vi "Get Helium Level.vi"(8 "error in (no error)":errorcluster, 11 "instrument.PPMS in":refnum<class "instrument.PPMS1.lvclass">) -> (0 "error out":errorcluster, 2 "LHe Level (%)":dbl, 3 "instrument.PPMS out":refnum<class "instrument.PPMS1.lvclass">)   [LabVIEW 2016, in "instrument.PPMS1.lvclass"]
uses:
  instrument.PPMS1.lvclass
  Typedefs/PPMS1.Commands-enum.ctl
panel:
  in  "Data":variant
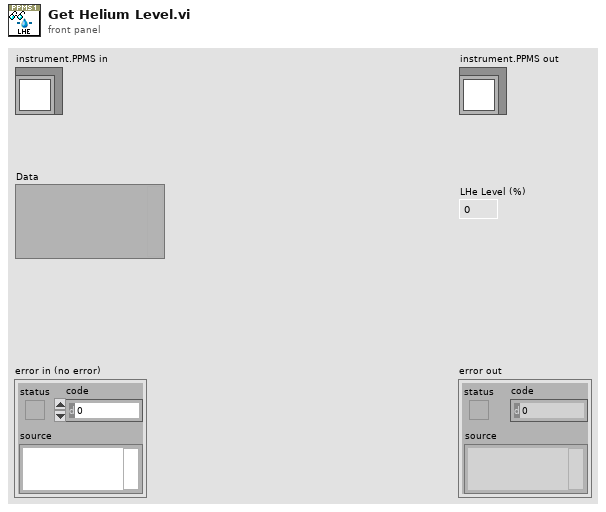
[diagram p1: front panel]
types:
  T1 = typedef "instrument.PPMS1.lvclass/PPMS1.Commands-enum.ctl" = enum16{"Get Magnet Field", "Get Helium Level", "Get Temperature", "Set Magnet Field", "Set Temperature", "getAll"}
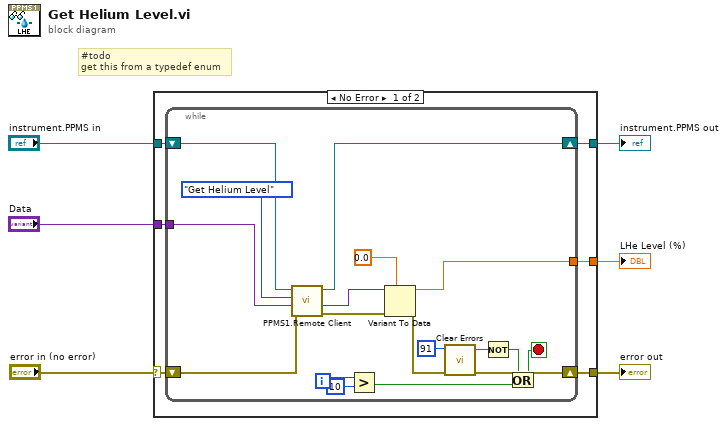
[diagram p0: block diagram]
diagram:
  # "#todo\nget this from a typedef enum"
  n1 = case shown="No Error" "error in (no error)" {
    selector: "error in (no error)" -> [w9 w32]
    tunnel: [w7 _] -> w6
    tunnel: "Data" -> [w12 _]
    tunnel: "instrument.PPMS in" -> [w11 w31]
    tunnel: [w8 w32] -> w3
    tunnel: [w10 w31] -> w2
    frame No Error {
      n2 = while {
        tunnel: w12 -> [w28]
        tunnel: [w19] -> w7
        shift-right: [w23] -> w10
        shift-left: w11 -> [w25]
        shift-right: [w21] -> w8
        shift-left: w9 -> [w22]
        i -> [w17]
        stop <- w15 stop-if-true
        n3 = call "PPMS1.Remote Client.vi"("error in (no error)"=w22, "Data"=w28, "Command"=PPMS1.Commands-enum."Get Helium Level", "instrument.PPMS in"=w25) -> ("error out"=w29:errorcluster, "Data out"=w26:variant, "instrument.PPMS out"=w23:refnum<class "instrument.PPMS1.lvclass">)  [unwired: 4 in, 1 out]
        n4 = Greater?(x=w17, y=10) -> (0:w13:bool)
        n5 = Variant To Data(error in=w29, type=0.0, Variant=w26) -> (data=w19:dbl, error out=w24:errorcluster)
        n6 = call <vilib>:"Clear Errors.vi"("error in (no error)"=w24, "specific error code to clear (0: all)"=91) -> ("error out"=w21:errorcluster, "specific error cleared?"=w18:bool)  [unwired: 4 in]
        n7 = Not(x=w18) -> (.not. x?=w14:bool)
        n8 = Or(x=w14, y=w13) -> (x .or. y?=w15:bool)
      }
    }
    frame Error {
    }
  }
  "error out" <- w3
  "instrument.PPMS out" <- w2
  "LHe Level (%)" <- w6
